vi "SanePressureCull.vi"(8 "GoodPressureXvals":i32[](array[numeric]), 10 "DataIn":T1) -> (2 "DataOut":T1)   [LabVIEW 2016]
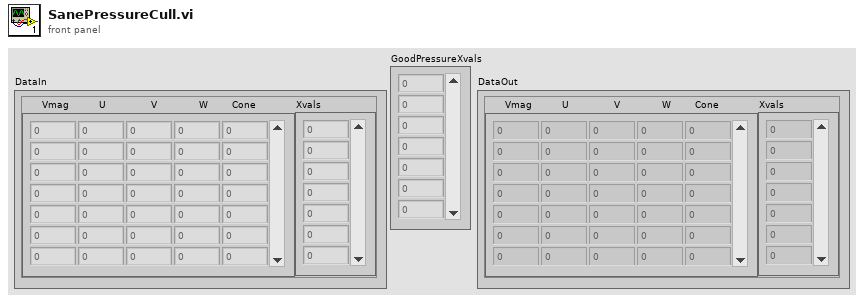
[diagram p1: front panel]
types:
  T1 = cluster{"   Vmag          U               V              W        Cone":dbl[][], "Xvals":i32[]}
  T2 = cluster{"   Vmag          U               V              W        Cone":dbl[][], i32[]}
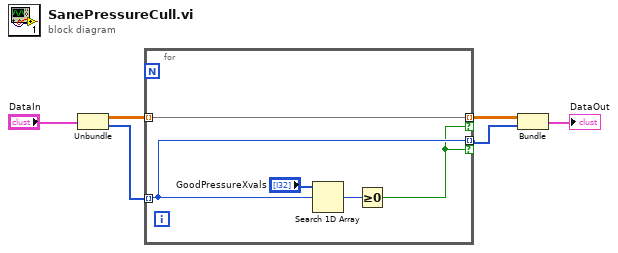
[diagram p0: block diagram]
diagram:
  n1 = Unbundle("DataIn") -> ("Vmag          U               V              W        Cone"=w5:dbl[][], "Xvals"=w4:i32[])
  n2 = for {
    tunnel: w5 -> [w9] mode=indexing
    tunnel: w4 -> [w8] mode=indexing
    tunnel: [w9] -> w3 mode=indexing if=w7
    tunnel: [w8] -> w2 mode=indexing if=w7
    n3 = Search 1D Array(1D array="GoodPressureXvals", element=w8) -> (index of element=w10:i32)  [unwired: 1 in]
    n4 = Greater Or Equal To 0?(x=w10) -> (x >= 0?=w7:bool)
  }
  n5 = Bundle("Vmag          U               V              W        Cone"=w3, w2) -> (→"DataOut":T2)  [unwired: 1 in]
